vi "Update PID Parameters Listbox.vi"(10 "Gain Schedule":T1(array[cluster]), 11 "MulticolumnListbox in":refnum<vi>) -> (3 "MulticolumnListbox out":refnum<vi>)   [LabVIEW 2019, in "PID Control Workspace Tool.lvlib"]
uses:
  PID Control Workspace Tool.lvlib
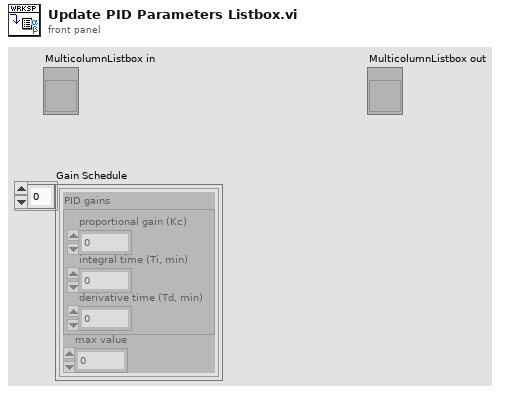
[diagram p1: front panel]
types:
  T1 = cluster{"PID gains":cluster{"proportional gain (Kc)":dbl, "integral time (Ti, min)":dbl, "derivative time (Td, min)":dbl}, "max value":dbl}[]
  T2 = cluster{"proportional gain (Kc)":dbl, "integral time (Ti, min)":dbl, "derivative time (Td, min)":dbl}
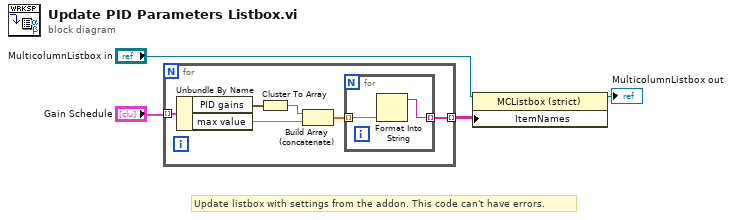
[diagram p0: block diagram]
diagram:
  # "Update listbox with settings from the addon. This code can't have errors."
  n1 = for {
    tunnel: "Gain Schedule" -> [w10] mode=indexing
    tunnel: [w9] -> w2 mode=indexing
    n2 = Unbundle By Name(w10) -> ("PID gains"=w8:T2, "max value"=w5:dbl)
    n3 = Cluster To Array(cluster=w8) -> (array=w7:dbl[])
    n4 = Build Array (concatenate)(w7, w5) -> (w6:dbl[])
    n5 = for {
      tunnel: w6 -> [w11] mode=indexing
      tunnel: [w12] -> w9 mode=indexing
      n6 = Format Into String(w11) -> (resulting string=w12:string)  [unwired: 3 in, 1 out]
    }
  }
  n7 = property class="MCListbox (strict)"(reference="MulticolumnListbox in", "ItemNames"=w2) -> (reference out=→"MulticolumnListbox out":refnum<vi>)  [unwired: 1 in, 1 out]
